vi "Close.vi"(8 "error in (no error)":errorcluster, 11 "Parallax PING))) in":refnum<class "Parallax PING))).lvclass">) -> (0 "error out":errorcluster)   [LabVIEW 2013, in "Parallax PING))).lvclass"]
doc: "Terminates the software connection to the sensor."
uses:
  Parallax PING))).lvclass
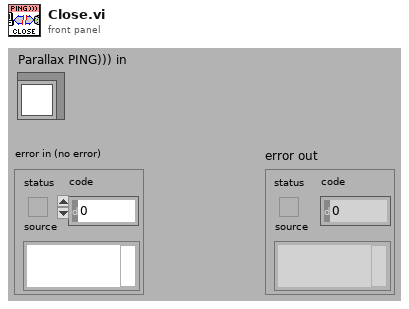
[diagram p1: front panel]
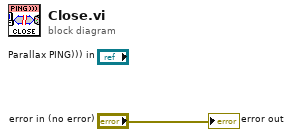
[diagram p0: block diagram]
diagram:
  "error out" <- "error in (no error)"
